vi "UnloadGraphWin.vi"(8 "error in (no error)":errorcluster caption="entrée d'erreur (pas d'erreur)", 11 "Interface en entrée":refnum<class "Interface.lvclass"> caption="DNL_LabVIEW Object in") -> (0 "error out":errorcluster caption="sortie d'erreur", 3 "Interface en sortie":refnum<class "Interface.lvclass"> caption="DNL_LabVIEW Object out")   [LabVIEW 2010, in "Interface.lvclass"]
uses:
  Interface.lvclass
  Interface.lvclass/Interface.ctl
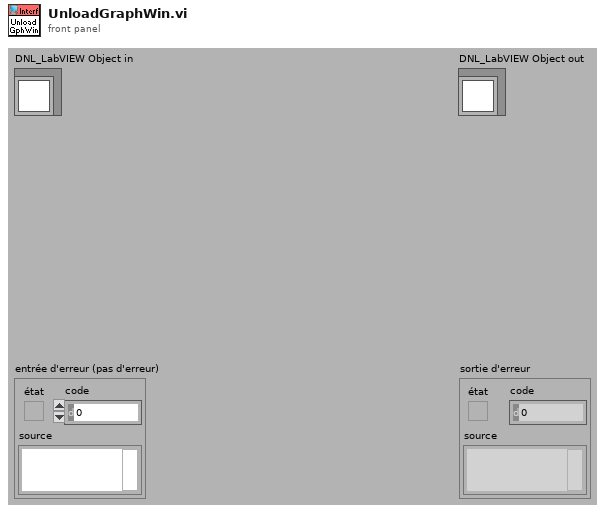
[diagram p1: front panel]
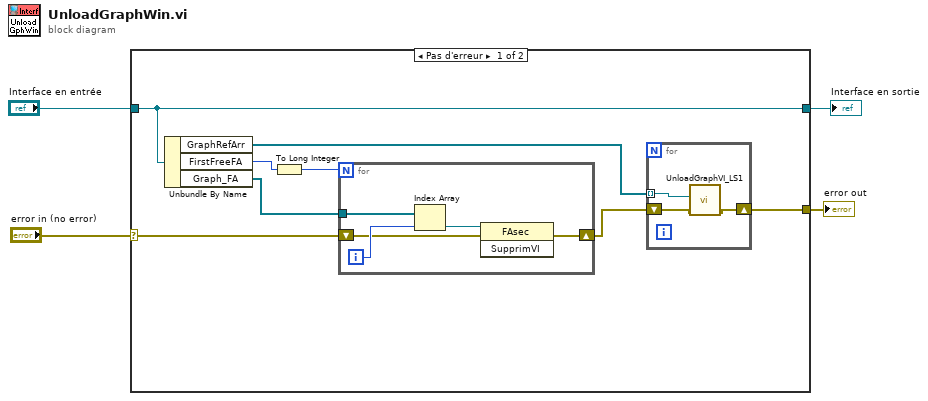
[diagram p0: block diagram]
diagram:
  n1 = case shown="Pas d'erreur" "error in (no error)" {
    selector: "error in (no error)" -> [w9 w22]
    tunnel: [w11 w22] -> w3
    tunnel: [w12 w21] -> w1
    tunnel: "Interface en entrée" -> [w12 w21]
    frame No Error {
      n2 = Unbundle By Name(w12) -> ("GraphRefArr"=w6:refnum<vi>[], "FirstFreeFA"=w7:u8, "Graph_FA"=w8:refnum<vi>[])
      n3 = To Long Integer(number=w7) -> (32bit integer=w10:i32)
      n4 = for {
        N: w10 -> [_]
        tunnel: w8 -> [w17]
        shift-right: [w13] -> w5
        shift-left: w9 -> [w14]
        i -> [w16]
        n5 = Index Array(array=w17, index=w16) -> (element=w15:refnum<vi>)
        n6 = invoke class="FAsec" method="SupprimVI"(reference=w15, error in=w14) -> (error out=w13:errorcluster)  [unwired: 1 in, 2 out]
      }
      n7 = for {
        tunnel: w6 -> [w20] mode=indexing
        shift-right: [w18] -> w11
        shift-left: w5 -> [w19]
        n8 = call "UnloadGraphVI_LS1.vi"("ErrorIn(No Error)"=w19, "GraphRef"=w20) -> ("sortie d'erreur"=w18:errorcluster)  [unwired: 9 in]
      }
    }
    frame Error {
    }
  }
  "error out" <- w3
  "Interface en sortie" <- w1
